vi "ELVIS III v1.0 Reserve DI Block.vi"(7 "Allow multiple opens?":bool, 8 "error in (no error)":errorcluster, 10 "DI (N Samples) Channel List":T2, 11 "Generic FPGA Reference":T1) -> (0 "error out":errorcluster)   [LabVIEW 2021]
uses:
  <vilib>/myRIO/Common/Instrument Driver Framework/myRIO v1.0/DI Block/typedefs/DI Block Channels List.ctl
  <vilib>/myRIO/Common/Instrument Driver Framework/myRIO v1.0/DI Block/typedefs/DI Block Channels Enum.ctl
  <vilib>/myRIO/Common/Instrument Driver Framework/Utilities/typedefs/Generic FPGA Reference.ctl
  <vilib>/myRIO/Common/Instrument Driver Framework/ELVIS III v1.0/Resource Manager/vis/ELVIS III v1.0 Create Configuration List.vi
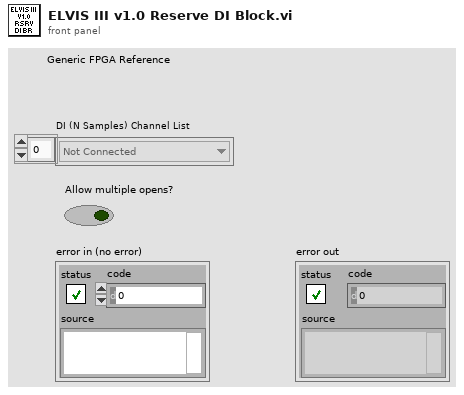
[diagram p1: front panel]
types:
  T1 = typedef "Generic FPGA Reference.ctl" = refnum<k20>
  T2 = typedef "DI Block Channels List.ctl" = T3[]
  T3 = typedef "DI Block Channels Enum.ctl" = enum16{"Not Connected", "A/DI0 (N Samples)", "A/DI1 (N Samples)", "A/DI2 (N Samples)", "A/DI3 (N Samples)", "A/DI4 (N Samples)", "A/DI5 (N Samples)", "A/DI6 (N Samples)", "A/DI7 (N Samples)", "A/DI8 (N Samples)", "A/DI9 (N Samples)", "A/DI10 (N Samples)", "A/DI11 (N Samples)", "A/DI12 (N Samples)", "A/DI13 (N Samples)", "A/DI14 (N Samples)", "A/DI15 (N Samples)", "A/DI16 (N Samples)", "A/DI17 (N Samples)", "A/DI18 (N Samples)", "A/DI19 (N Samples)", "B/DI0 (N Samples)", "B/DI1 (N Samples)", "B/DI2 (N Samples)", "B/DI3 (N Samples)", "B/DI4 (N Samples)", "B/DI5 (N Samples)", "B/DI6 (N Samples)", "B/DI7 (N Samples)", "B/DI8 (N Samples)", "B/DI9 (N Samples)", "B/DI10 (N Samples)", "B/DI11 (N Samples)", "B/DI12 (N Samples)", "B/DI13 (N Samples)", "B/DI14 (N Samples)", "B/DI15 (N Samples)", "B/DI16 (N Samples)", "B/DI17 (N Samples)", "B/DI18 (N Samples)", "B/DI19 (N Samples)"}
  T4 = typedef "ELVIS III v1.0 Channel Reservation List.ctl" = T5[]
  T5 = typedef "ELVIS III v1.0 Channel Reservation Info.ctl" = cluster{"Channel Name":string, "Connector":T6, "MutexIDs":u32[]}
  T6 = typedef "ELVIS III v1.0 Connector List.ctl" = enum32{"None", "ConnectorA", "ConnectorB"}
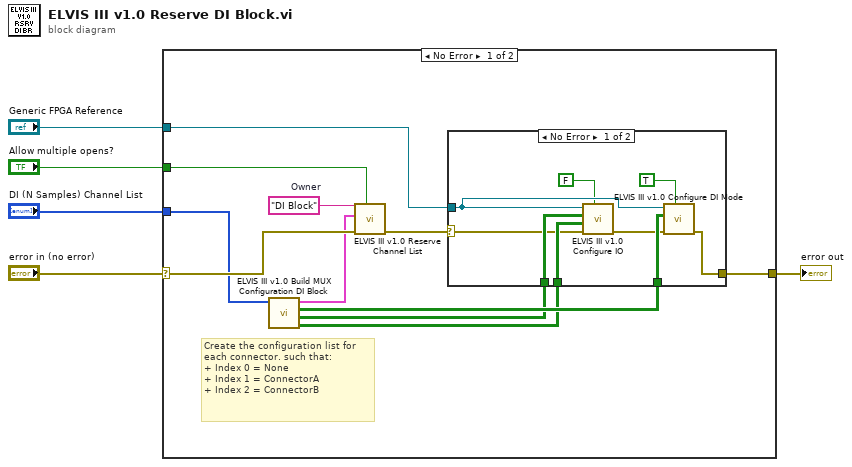
[diagram p0: block diagram]
diagram:
  n1 = case shown="No Error" "error in (no error)" {
    selector: "error in (no error)" -> [w15 w27]
    tunnel: "DI (N Samples) Channel List" -> [w12 _]
    tunnel: [w8 w27] -> w4
    tunnel: "Allow multiple opens?" -> [w16 _]
    tunnel: "Generic FPGA Reference" -> [w10 _]
    frame No Error {
      w14 = "DI Block"  # Owner
      # "Create the configuration list for each connector. such that:\n+ Index 0 = None\n+ Index 1 = ConnectorA\n+ Index 2 = ConnectorB"
      n2 = call <vilib>:"ELVIS III v1.0 Build MUX Configuration DI Block.vi"("DI (N Samples) Channel List"=w12) -> ("Configuration Bitmask Array"=w6:bool[][], "Configration Bitcode Array"=w7:bool[][], "DIO Mode Bitask"=w9:bool[][], "Channel Reservation List"=w13:T4)  [unwired: 7 in]
      n3 = call <vilib>:"ELVIS III v1.0 Reserve Channel List.vi"("Allow multiple opens?"=w16, "error in (no error)"=w15, "Channel Reservation List"=w13, "Owner"=w14) -> ("error out"=w11:errorcluster)  [unwired: 7 in]
      n4 = case shown="No Error" w11 {
        selector: w11 -> [w20 w26]
        tunnel: w10 -> [w18 _]
        tunnel: w9 -> [w25 _]
        tunnel: [w23 w26] -> w8
        tunnel: w7 -> [w22 _]
        tunnel: w6 -> [w21 _]
        frame No Error {
          n5 = call <vilib>:"ELVIS III v1.0 Configure IO.vi"("Value"=FALSE, "error in (no error)"=w20, "Bitmask Array"=w21, "Bitcode Array"=w22, "myRIO FPGA Ref In"=w18) -> ("error out"=w19:errorcluster)  [unwired: 6 in]
          n6 = call <vilib>:"ELVIS III v1.0 Configure DI Mode.vi"("Apply Bitmask?"=TRUE ("Set or Reset?"), "error in (no error)"=w19, "Bitmask Array"=w25, "myRIO FPGA Ref In"=w18) -> ("error out"=w23:errorcluster)  [unwired: 7 in]
        }
        frame Error {
        }
      }
    }
    frame Error {
    }
  }
  "error out" <- w4
